vi "add_alignment_rings.vi"(4 "Color":u32(colorbox)=16448250, 5 "number of rings":i32, 9 "Image in":T1) -> (3 "Image Out":T1)   [LabVIEW 2011]
uses:
  <vilib>/vision/Image Controls.llb/IMAQ Image.ctl
  global_vars.vi
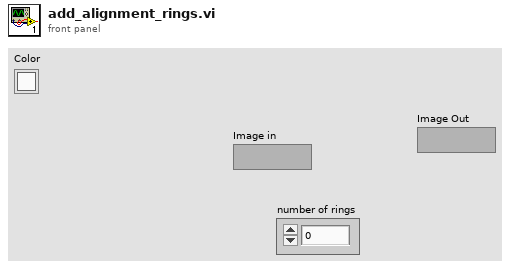
[diagram p1: front panel]
types:
  T1 = typedef "IMAQ Image.ctl" = refnum<image>
  T2 = cluster{"Numeric Control":dbl, "Numeric Control":dbl, "Numeric Control":dbl, "Numeric Control":dbl}
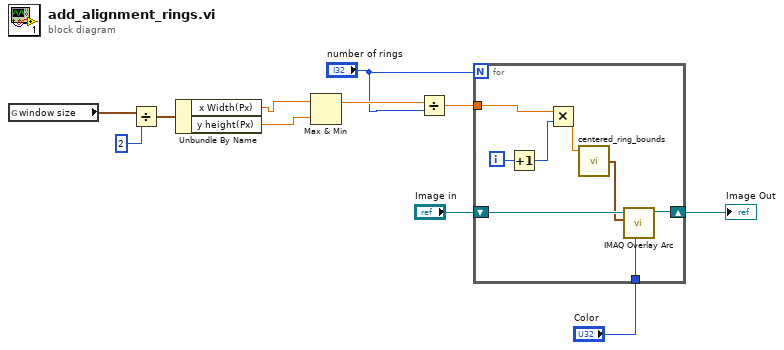
[diagram p0: block diagram]
diagram:
  n1 = global read "global_vars.vi" "window size"() -> (w10:cluster{"x Width(Px)":i32, "y height(Px)":i32})
  n2 = Divide(x=w10, y=2 ("y height(Px)")) -> (x/y=w9:cluster{"x Width(Px)":dbl, "y height(Px)":dbl})
  n3 = Unbundle By Name(w9) -> ("x Width(Px)"=w8:dbl, "y height(Px)"=w7:dbl)
  n4 = Max & Min(x=w8, y=w7) -> (max(x,y)=w6:dbl)  [unwired: 1 out]
  n5 = Divide(x=w6, y="number of rings") -> (x/y=w5:dbl)
  n6 = for {
    N: "number of rings" -> [_]
    shift-right: [w13] -> w2
    shift-left: "Image in" -> [w19]
    tunnel: w5 -> [w16]
    tunnel: "Color" -> [w12]
    i -> [w17]
    n7 = Increment(x=w17) -> (x+1=w15:i32)
    n8 = Multiply(x=w16, y=w15) -> (x*y=w18:dbl)
    n9 = call "centered_ring_bounds.vi"("radius R"=w18) -> ("Bounding Rectangle"=w14:T2)  [unwired: 4 in]
    n10 = call "IMAQ Overlay Arc"("Color"=w12, "Bounding Rectangle"=w14, "Image"=w19) -> ("Image Out"=w13:T1)  [unwired: 7 in, 1 out]
  }
  "Image Out" <- w2
